vi "Get FOV and Phi.vi"(0 "Distance [um]":dbl, 3 "Transformation Matrix":T1, 5 "Initial [pix]":cluster{"X":i32, "Y":i32}, 7 "Final [pix]":cluster{"X":i32, "Y":i32}, 9 "Image Size [pix]":cluster{"Width":u32, "Height":u32}) -> (4 "FOV [um]":cluster{"Width":dbl, "Height":dbl}, 6 "Angle [rad]":dbl)   [LabVIEW 2012, in "Targeting Unit.lvlib"]
uses:
  <vilib>/Analysis/Matrix/Datatypes/RealMatrix.ctl
  Targeting Unit.lvlib
  <vilib>/Analysis/Matrix/NI_Matrix.lvlib
panel:
  # "X entering (1) or exiting tip (-1)"
  # "Flip (Yes -1 No 1)"
  # "Insertion step coefficient"
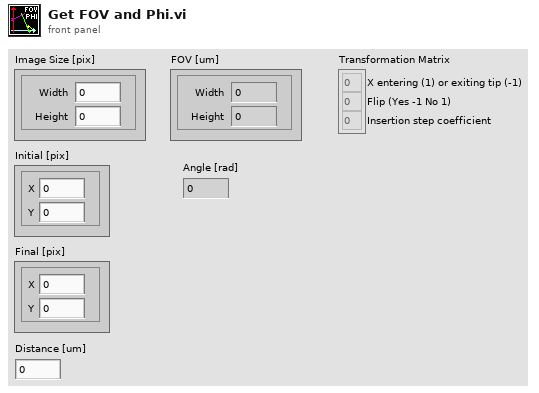
[diagram p1: front panel]
types:
  T1 = typedef "NI_Matrix.lvlib/RealMatrix.ctl" = dbl[][]
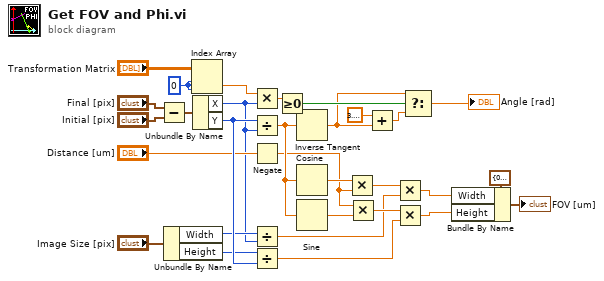
[diagram p0: block diagram]
diagram:
  w3 = 0 ("index (row)")
  n1 = Subtract(x="Final [pix]", y="Initial [pix]") -> (x-y=w16:cluster{"X":i32, "Y":i32})
  n2 = Unbundle By Name("Image Size [pix]") -> ("Width"=w11:u32, "Height"=w10:u32)
  n3 = Index Array(array="Transformation Matrix", index (row)=w3, index (col)=w3) -> (element=w1:dbl)
  n4 = Unbundle By Name(w16) -> ("X"=w4:i32, "Y"=w15:i32)
  n5 = Multiply(x=w1, y=w4) -> (x*y=w5:dbl)
  n6 = Divide(x=w15, y=w4) -> (x/y=w20:dbl)
  n7 = Negate(x="Distance [um]") -> (-x=w19:dbl)
  n8 = Divide(x=w11, y=w4) -> (x/y=w27:dbl)
  n9 = Divide(x=w10, y=w15) -> (x/y=w26:dbl)
  n10 = Greater Or Equal To 0?(x=w5) -> (x >= 0?=w23:bool)
  n11 = Inverse Tangent(1:w20) -> (0:w22:dbl)
  n12 = Cosine(x=w20) -> (cos(x)=w25:dbl)
  n13 = Sine(x=w20) -> (sin(x)=w30:dbl)
  n14 = Multiply(x=w25, y=w19) -> (x*y=w29:dbl)
  n15 = Multiply(x=w19, y=w30) -> (x*y=w28:dbl)
  n16 = Add(x=3.141592653589793, y=w22) -> (x+y=w24:dbl)
  n17 = Multiply(x=w29, y=w27) -> (x*y=w6:dbl)
  n18 = Multiply(x=w28, y=w26) -> (x*y=w7:dbl)
  n19 = Select(t=w22, s=w23, f=w24) -> (s? t:f=→"Angle [rad]":dbl)
  n20 = Bundle By Name(cluster=cluster{"Width":dbl, "Height":dbl} {"Width"=0.0, "Height"=0.0} ("FOV [um]"), "Width"=w6, "Height"=w7) -> (→"FOV [um]":cluster{"Width":dbl, "Height":dbl})
